vi "Host_SetParameters_new.vi"() -> ()   [LabVIEW 2018]
uses:
  Master/TypeDef_LoopPeriods.ctl
  Type_Def/TypeDef_LoopPeriod.ctl
panel:
  in  "Nav Period (ms)":u32=10
  in  "CAN Period (ms)":i64=90
  in  "IMU Period (ms)":u32=5
  in  "DAQ Period (ms)":u32=100
  in  "Control Period (ms)":i64=10
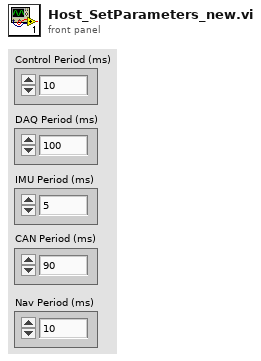
[diagram p1: front panel]
types:
  T1 = typedef "TypeDef_LoopPeriods.ctl" = cluster{"Control Period":i64, "DAQ Period":u32, "IMU Period":u32, "CAN Period":i64, "Nav Period":u32}
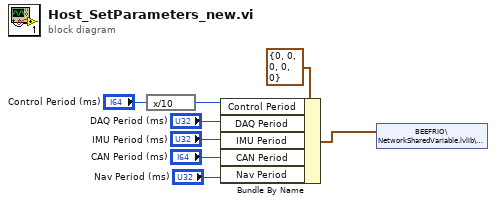
[diagram p0: block diagram]
diagram:
  n1 = expression code="x/10"("Control Period (ms)") -> (w7:i64)
  n2 = Bundle By Name(cluster=T1 {"Control Period"=0, "DAQ Period"=0, "IMU Period"=0, "CAN Period"=0, "Nav Period"=0} ("input cluster"), "Control Period"=w7, "DAQ Period"="DAQ Period (ms)", "IMU Period"="IMU Period (ms)", "CAN Period"="CAN Period (ms)", "Nav Period"="Nav Period (ms)") -> (w8:T1)
  n3 = shared-variable "BEEFRIO\\NetworkSharedVariable.lvlib\\LoopPeriods"(w8) -> ()  [unwired: 1 in, 1 out]
